vi "Set Settings.vi"(8 "error in (no error)":errorcluster, 10 "Settings":T1, 11 "Temp01 in":refnum<class "TELLC_Temp01.lvclass">) -> (0 "error out":errorcluster, 3 "Temp01 out":refnum<class "TELLC_Temp01.lvclass">)   [LabVIEW 2017, in "TELLC_Temp01.lvclass"]
doc: "Developed by Kevin Thompson\nkevin@thompsonengineering.net\n\nCopyright 2018\nThompson Engineering, LLC"
uses:
  TELLC_Temp01.lvclass
  DataTypes/Settings--cluster.ctl
  TELLC_Temp01.lvclass/TELLC_Temp01.ctl
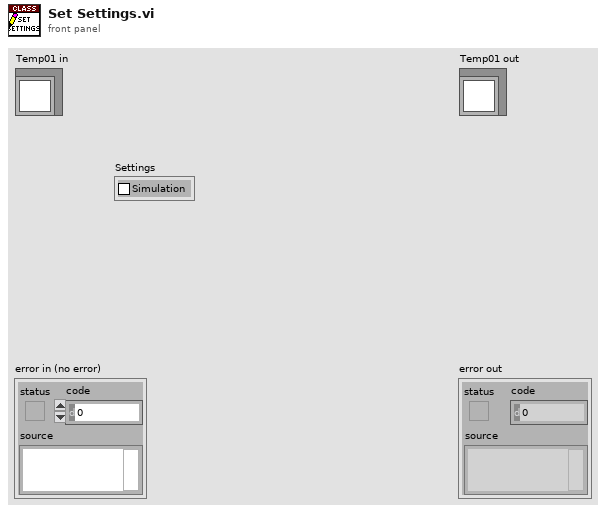
[diagram p1: front panel]
types:
  T1 = typedef "TELLC_Temp01.lvclass/Settings--cluster.ctl" = cluster{"Simulation":bool}
  T2 = typedef "TELLC_Temp01.lvclass/ObjData--cluster.ctl" = cluster{"Settings":T1, "ReadData-placeholder":T3, "VISA-placeholder":refnum<visa-resource-name>}
  T3 = typedef "TELLC_Temp01.lvclass/Read Data--cluster.ctl" = cluster{"Data":dbl}
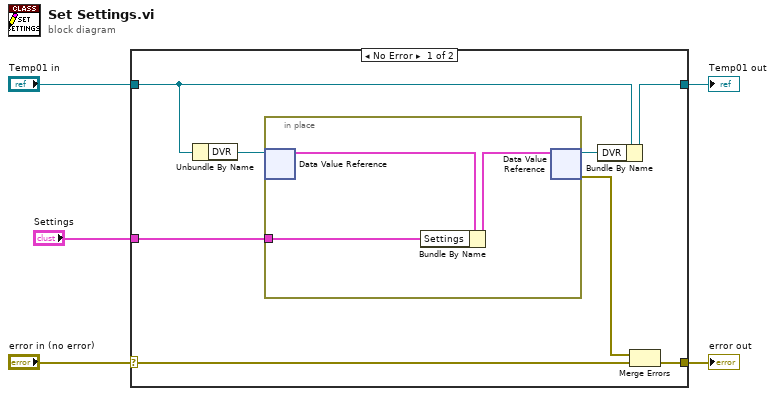
[diagram p0: block diagram]
diagram:
  n1 = case shown="No Error" "error in (no error)" {
    selector: "error in (no error)" -> [w13 w17]
    tunnel: [w8 w17] -> w4
    tunnel: [w9 w18] -> w2
    tunnel: "Temp01 in" -> [w12 w18]
    tunnel: "Settings" -> [w6 _]
    frame No Error {
      n2 = Unbundle By Name(w12) -> ("DVR"=w11:refnum<data-value>)
      n3 = in-place {
        in-place-border: w6 -> [w14]
        n4 = in-place-dvr #1(w11) -> (w16:T2)  [unwired: 1 out]
        n5 = Bundle By Name(cluster=w16, "Settings"=w14) -> (w15:T2)
        n6 = in-place-dvr #1(w15) -> (w10:refnum<data-value>, w7:errorcluster)
      }
      n7 = Bundle By Name(cluster=w12, "DVR"=w10) -> (w9:refnum<class "TELLC_Temp01.lvclass">)
      n8 = Merge Errors(w7, w13) -> (w8:errorcluster)
    }
    frame Error {
    }
  }
  "error out" <- w4
  "Temp01 out" <- w2
